vi "multiplex_controller.vi"() -> ()   [LabVIEW 2013]
uses:
  <instrlib>/lv70drivers/srsQcm200lv7drivers.llb/DialogType.ctl
  <vilib>/DAQmx/write.llb/DAQmx Write (Digital 1D Bool 1Chan 1Samp).vi
  <vilib>/DAQmx/create/channels.llb/DAQmx Create Channel (DO-Digital Output).vi
  <vilib>/DAQmx/miscellaneous.llb/DAQmx Fill In Error Info.vi
panel:
  out "Current Channel\nEnabled":dbl
  in  "Enable Channel":T1(ring)
  in  "Stop 2":bool
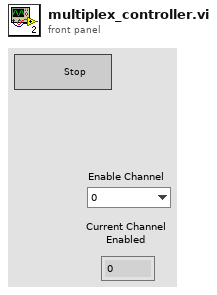
[diagram p1: front panel]
types:
  T1 = enum16{"0", "1", "2", "3", "4", "5", "6", "7", "8", "9", "10", "11", "12", "13", "14", "15"}
  T2 = typedef "DialogType.ctl" = u16
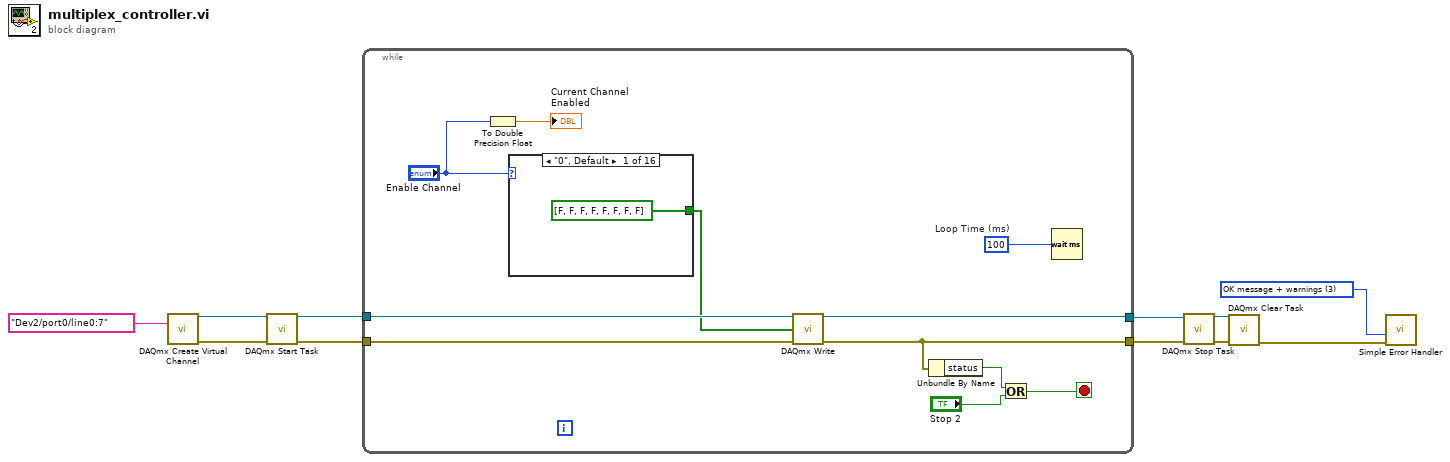
[diagram p0: block diagram]
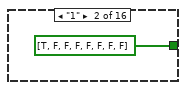
[diagram p2: hidden frame]
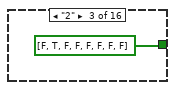
[diagram p3: hidden frame]
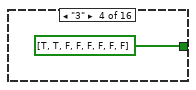
[diagram p4: hidden frame]
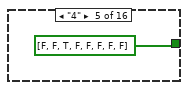
[diagram p5: hidden frame]
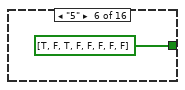
[diagram p6: hidden frame]
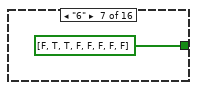
[diagram p7: hidden frame]
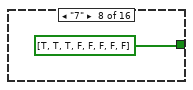
[diagram p8: hidden frame]
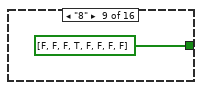
[diagram p9: hidden frame]
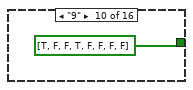
[diagram p10: hidden frame]
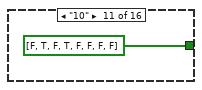
[diagram p11: hidden frame]
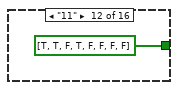
[diagram p12: hidden frame]
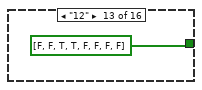
[diagram p13: hidden frame]
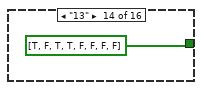
[diagram p14: hidden frame]
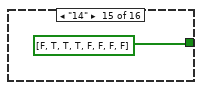
[diagram p15: hidden frame]
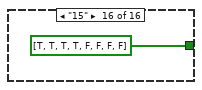
[diagram p16: hidden frame]
diagram:
  w5 = T2 3 items=["no dialog", "OK message", "continue or stop message", "OK message + warnings", "continue/stop + warnings"] ("type of dialog (OK msg:1)")
  n1 = call-poly <vilib>:"DAQmx Create Virtual Channel.vi"("lines"=tag "Dev2/port0/line0:7" ("Line(s)")) -> ("task out"=w8:refnum<k21>, "error out"=w9:errorcluster)  [unwired: 13 in]
  n2 = call <vilib>:"DAQmx Start Task.vi"("task/channels in"=w8, "error in"=w9) -> ("task out"=w4:refnum<k21>, "error out"=w3:errorcluster)  [unwired: 12 in]
  n3 = while {
    tunnel: w4 -> [w18]
    tunnel: w3 -> [w17]
    tunnel: [w16] -> w2
    tunnel: [w15] -> w1
    stop <- w19 stop-if-true
    w22 = u32 100  # Loop Time (ms)
    n4 = To Double Precision Float(number="Enable Channel") -> (double precision float=→"Current Channel\nEnabled":dbl)
    n5 = case shown="\"0\", Default" "Enable Channel" {
      tunnel: [bool[] [FALSE, FALSE, FALSE, FALSE, FALSE, FALSE, FALSE, FALSE] ("Output Array") bool[] [TRUE, FALSE, FALSE, FALSE, FALSE, FALSE, FALSE, FALSE] ("Output Array") bool[] [FALSE, TRUE, FALSE, FALSE, FALSE, FALSE, FALSE, FALSE] ("Output Array") bool[] [TRUE, TRUE, FALSE, FALSE, FALSE, FALSE, FALSE, FALSE] ("Output Array") bool[] [FALSE, FALSE, TRUE, FALSE, FALSE, FALSE, FALSE, FALSE] ("Output Array") bool[] [TRUE, FALSE, TRUE, FALSE, FALSE, FALSE, FALSE, FALSE] ("Output Array") bool[] [FALSE, TRUE, TRUE, FALSE, FALSE, FALSE, FALSE, FALSE] ("Output Array") bool[] [TRUE, TRUE, TRUE, FALSE, FALSE, FALSE, FALSE, FALSE] ("Output Array") bool[] [FALSE, FALSE, FALSE, TRUE, FALSE, FALSE, FALSE, FALSE] ("Output Array") bool[] [TRUE, FALSE, FALSE, TRUE, FALSE, FALSE, FALSE, FALSE] ("Output Array") bool[] [FALSE, TRUE, FALSE, TRUE, FALSE, FALSE, FALSE, FALSE] ("Output Array") bool[] [TRUE, TRUE, FALSE, TRUE, FALSE, FALSE, FALSE, FALSE] ("Output Array") bool[] [FALSE, FALSE, TRUE, TRUE, FALSE, FALSE, FALSE, FALSE] ("Output Array") bool[] [TRUE, FALSE, TRUE, TRUE, FALSE, FALSE, FALSE, FALSE] ("Output Array") bool[] [FALSE, TRUE, TRUE, TRUE, FALSE, FALSE, FALSE, FALSE] ("Output Array") bool[] [TRUE, TRUE, TRUE, TRUE, FALSE, FALSE, FALSE, FALSE] ("Output Array")] -> w14
      frame "0", Default {
      }
      frame "1" {
      }
      frame "2" {
      }
      frame "3" {
      }
      frame "4" {
      }
      frame "5" {
      }
      frame "6" {
      }
      frame "7" {
      }
      frame "8" {
      }
      frame "9" {
      }
      frame "10" {
      }
      frame "11" {
      }
      frame "12" {
      }
      frame "13" {
      }
      frame "14" {
      }
      frame "15" {
      }
    }
    n6 = call-poly <vilib>:"DAQmx Write.vi"("task/channels in"=w18, "data"=w14, "error in"=w17) -> ("task out"=w15:refnum<k21>, "error out"=w16:errorcluster)  [unwired: 10 in, 1 out]
    n7 = Unbundle By Name(w16) -> ("status"=w20:bool)
    n8 = Or(x=w20, y="Stop 2") -> (x .or. y?=w19:bool)
    n9 = Wait (ms)(milliseconds to wait=w22) -> ()  [unwired: 1 out]
  }
  n10 = call <vilib>:"DAQmx Stop Task.vi"("task/channels in"=w1, "error in"=w2) -> ("task out"=w7:refnum<k21>, "error out"=w6:errorcluster)  [unwired: 12 in]
  n11 = call <vilib>:"DAQmx Clear Task.vi"("task in"=w7, "error in"=w6) -> ("error out"=w11:errorcluster)  [unwired: 13 in]
  n12 = call <vilib>:"Simple Error Handler.vi"("type of dialog (OK msg:1)"=w5, "error in (no error)"=w11) -> ()  [unwired: 3 in, 5 out]
